vi "get_single_acq.vi"(8 "error in (no error)":errorcluster, 11 "_cameraBase in":refnum<class "_cameraBase.lvclass">) -> (0 "error out":errorcluster, 1 "wavelengths":dbl[](array[numeric]), 2 "intensity":dbl[][](array[numeric]), 3 "_cameraBase out":refnum<class "_cameraBase.lvclass">, 4 "trig channel 2":bool[](array[boolean]), 6 "trig channel 1":bool[](array[boolean]))   [LabVIEW 2019, in "_cameraBase.lvclass"]
uses:
  _cameraBase.lvclass
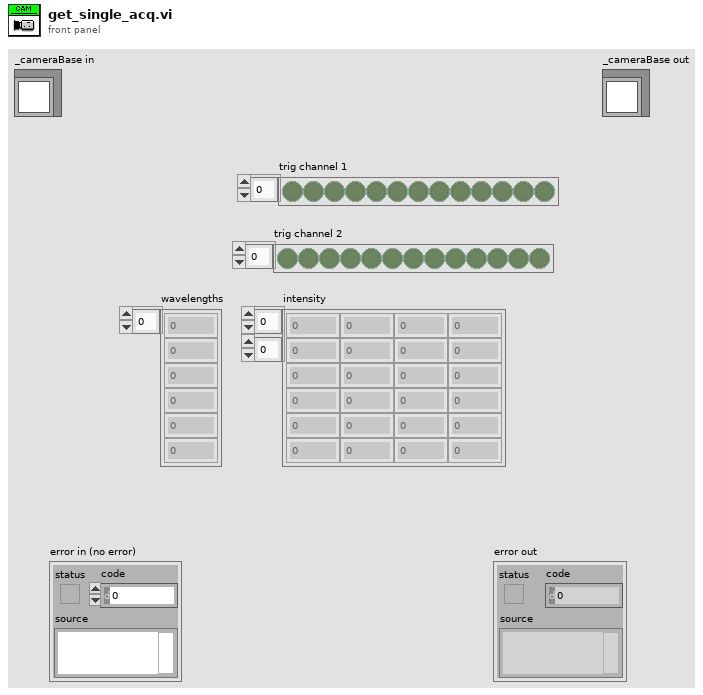
[diagram p1: front panel]
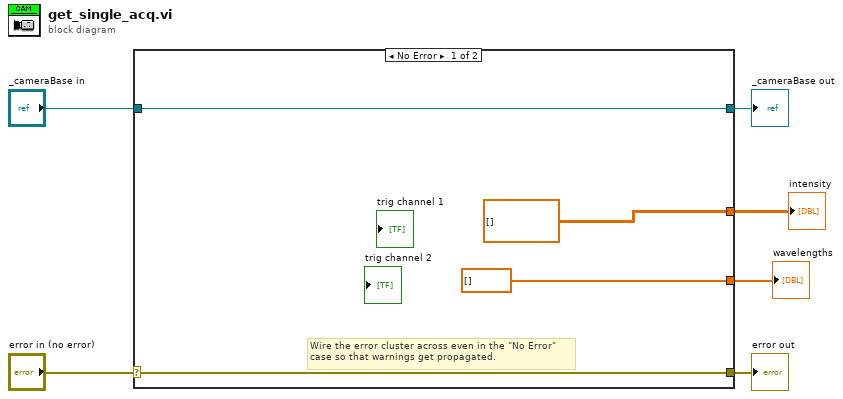
[diagram p0: block diagram]
diagram:
  n1 = case shown="No Error" "error in (no error)" {
    selector: "error in (no error)" -> [w9 w12]
    tunnel: [w9 w12] -> w5
    tunnel: [w10 w11] -> w3
    tunnel: "_cameraBase in" -> [w10 w11]
    tunnel: [dbl[][] [] ("Array") _] -> w2
    tunnel: [dbl[] [] ("wavelengths") _] -> w1
    frame No Error {
      # "Wire the error cluster across even in the \"No Error\"\ncase so that warnings get propagated."
    }
    frame Error {
    }
  }
  "error out" <- w5
  "_cameraBase out" <- w3
  "intensity" <- w2
  "wavelengths" <- w1
